vi "CC Script Parse Define Random Dither.vi"(8 "error in (no error)":errorcluster, 9 "To String?":bool, 10 "Random Dither in":T1={"Count"=1, "Radius"=1.0, "Name"=""}, 11 "Dither Parameters":string="\"Rnadome Dither Mispeller\" Count=3,Radius=1.23") -> (0 "error out":errorcluster, 2 "Random Dither out":T1={"Count"=1, "Radius"=1.0, "Name"=""}, 3 "Script String out":string="ObjectName \"RA\":\"123.456\",\"DEC\":\"4546.54\"")   [LabVIEW 2021]
uses:
  typedefs/CC cluster Random Dithering.ctl
  <vilib>/regexp/Match Regular Expression.xnode
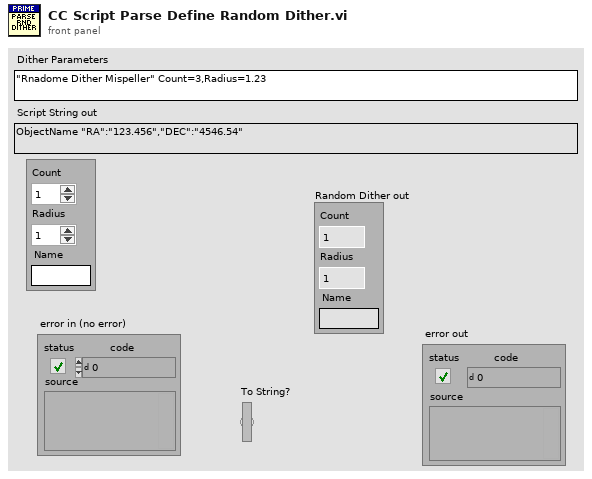
[diagram p1: front panel]
types:
  T1 = typedef "CC cluster Random Dithering.ctl" = cluster{"Count":i32, "Radius":dbl, "Name":string}
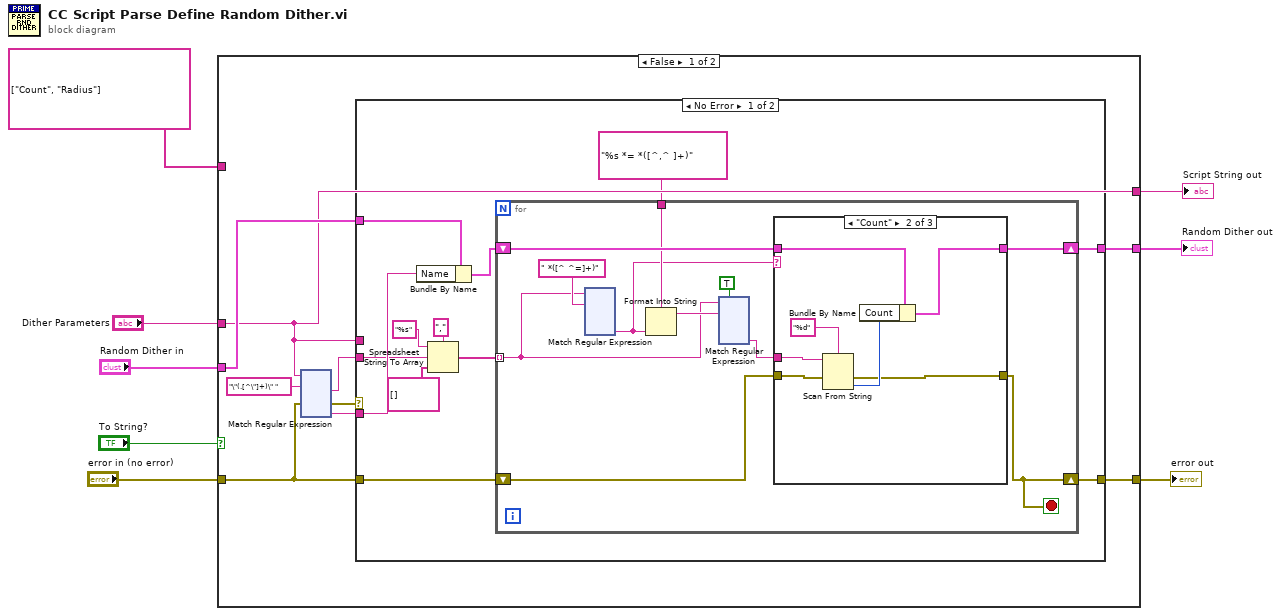
[diagram p0: block diagram]
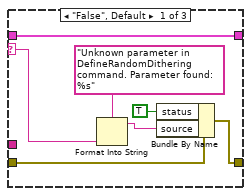
[diagram p2: hidden frame]
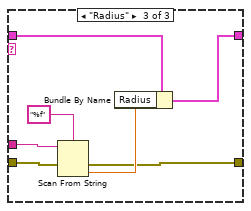
[diagram p3: hidden frame]
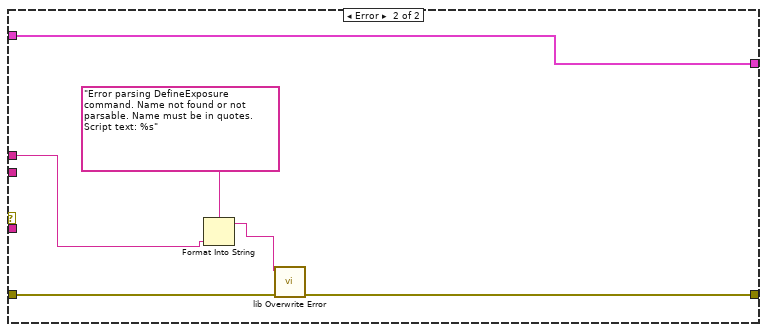
[diagram p4: hidden frame]
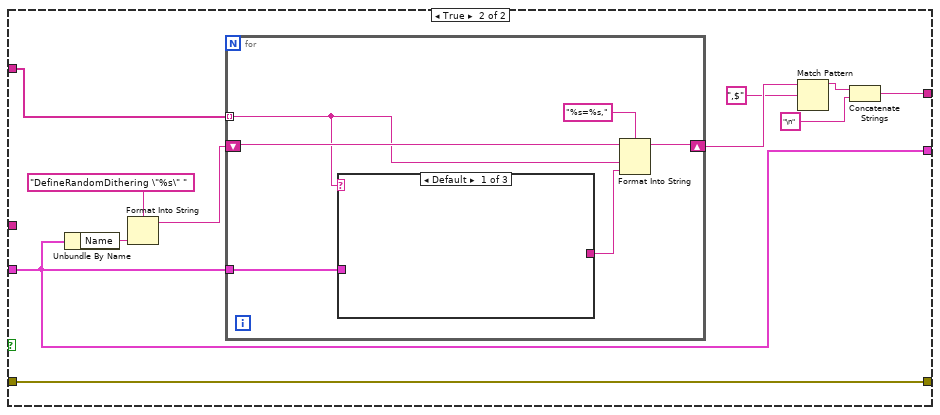
[diagram p5: hidden frame]
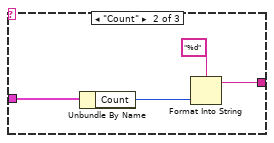
[diagram p6: hidden frame]
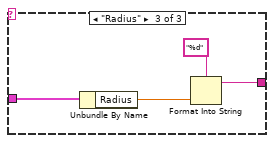
[diagram p7: hidden frame]
diagram:
  n1 = case shown="False" "To String?" {
    tunnel: "Dither Parameters" -> [w13 _]
    tunnel: string[] ["Count", "Radius"] -> [_ w431]
    tunnel: [w17 w427] -> w6
    tunnel: "error in (no error)" -> [w12 w430]
    tunnel: [w16 w430] -> w4
    tunnel: "Random Dither in" -> [w15 w427]
    tunnel: [w13 w429] -> w1
    frame False {
      n2 = xnode "Match Regular Expression"("input string"=w13, "regular expression"="\"(.[^\"]+)\" ", "error in"=w12) -> ("after match"=w9:string, "error out"=w11:errorcluster, "submatch 1"=w10:string)  [unwired: 3 in, 3 out]
      n3 = case shown="No Error" w11 {
        tunnel: [w148 w419] -> w17
        tunnel: [w147 w420] -> w16
        tunnel: w12 -> [w141 w421]
        tunnel: w13 -> [_ w423]
        tunnel: w15 -> [w139 w419]
        tunnel: w10 -> [w138 _]
        tunnel: w9 -> [w137 _]
        frame No Error {
          n4 = Bundle By Name(cluster=w139, "Name"=w138) -> (w140:T1)
          n5 = Spreadsheet String To Array(delimiter (Tab)=",", format string="%s", spreadsheet string=w137, array type (2D Dbl)=string[] []) -> (array=w143:string[])
          n6 = for {
            tunnel: w143 -> [w152] mode=indexing
            shift-right: [w158] -> w148
            shift-left: w140 -> [w159]
            shift-right: [w149] -> w147
            shift-left: w141 -> [w157]
            tunnel: "%s *= *([^,^ ]+)" ("regular expression") -> [w154]
            stop <- w149 stop-if-true
            n7 = xnode "Match Regular Expression"("input string"=w152, "regular expression"=" *([^ ^=]+)" ("format string")) -> ("submatch 1"=w151:string)  [unwired: 4 in, 5 out]
            n8 = Format Into String(format string=w154, w151) -> (resulting string=w156:string)  [unwired: 2 in, 1 out]
            n9 = xnode "Match Regular Expression"("input string"=w152, "regular expression"=w156, "ignore case? (F)"=TRUE) -> ("submatch 1"=w150:string)  [unwired: 3 in, 5 out]
            n10 = case shown="\"Count\"" w151 {
              selector: w151 -> [w402 _ _]
              tunnel: w159 -> [w404 w411 w418]
              tunnel: w150 -> [_ w409 w416]
              tunnel: [w404 w407 w415] -> w158
              tunnel: w157 -> [w401 w406 w413]
              tunnel: [w398 w405 w412] -> w149
              frame "False", Default {
                n11 = Format Into String(format string="Unknown parameter in DefineRandomDithering command. Parameter found: %s", w402) -> (resulting string=w400:string)  [unwired: 2 in, 1 out]
                n12 = Bundle By Name(cluster=w401, "status"=TRUE, "source"=w400) -> (w398:errorcluster)
              }
              frame "Count" {
                n13 = Scan From String(format string="%d", input string=w409, error in=w406) -> (error out=w405:errorcluster, output 1=w408:i32)  [unwired: 2 in, 2 out]
                n14 = Bundle By Name(cluster=w411, "Count"=w408) -> (w407:T1)
              }
              frame "Radius" {
                n15 = Scan From String(format string="%f", input string=w416, error in=w413) -> (error out=w412:errorcluster, output 1=w414:dbl)  [unwired: 2 in, 2 out]
                n16 = Bundle By Name(cluster=w418, "Radius"=w414) -> (w415:T1)
              }
            }
          }
        }
        frame Error {
          n17 = Format Into String(format string="Error parsing DefineExposure command. Name not found or not parsable. Name must be in quotes. Script text: %s", w423) -> (resulting string=w422:string)  [unwired: 2 in, 1 out]
          n18 = call "lib Overwrite Error.vi"("error in (no error)"=w421, "Error Message"=w422) -> ("error out"=w420:errorcluster)  [unwired: 9 in]
        }
      }
    }
    frame True {
      n19 = Unbundle By Name(w427) -> ("Name"=w426:string)
      n20 = Format Into String(format string="DefineRandomDithering \"%s\" ", w426) -> (resulting string=w425:string)  [unwired: 2 in, 1 out]
      n21 = for {
        tunnel: w431 -> [w438] mode=indexing
        shift-right: [w436] -> w435
        shift-left: w425 -> [w440]
        tunnel: w427 -> [w441]
        n22 = case shown="Default" w438 {
          tunnel: w441 -> [_ w445 w449]
          tunnel: [_ w442 w446] -> w437
          frame Default {
          }
          frame "Count" {
            n23 = Unbundle By Name(w445) -> ("Count"=w443:i32)
            n24 = Format Into String(format string="%d", w443) -> (resulting string=w442:string)  [unwired: 2 in, 1 out]
          }
          frame "Radius" {
            n25 = Unbundle By Name(w449) -> ("Radius"=w447:dbl)
            n26 = Format Into String(format string="%d", w447) -> (resulting string=w446:string)  [unwired: 2 in, 1 out]
          }
        }
        n27 = Format Into String(format string="%s=%s,", initial string=w440, w438, w437) -> (resulting string=w436:string)  [unwired: 1 in, 1 out]
      }
      n28 = Match Pattern(string=w435, regular expression=",$") -> (before substring=w433:string)  [unwired: 1 in, 3 out]
      n29 = Concatenate Strings(w433, "\n" ("string")) -> (w429:string)
    }
  }
  "error out" <- w4
  "Random Dither out" <- w6
  "Script String out" <- w1
